vi "Open Project Reference.vi"(8 "error in (no error)":errorcluster, 10 "Path":path, 11 "App Ref":refnum<vi>) -> (0 "error out":errorcluster, 2 "VI Server Configured?":bool, 3 "App Ref out":refnum<vi>)   [LabVIEW 2020, in "MacroAssert.lvlib"]
doc: "Opens and outputs an application reference to a development system application instance that is owned by the project at <B>Path</B>."
uses:
  MacroAssert.lvlib
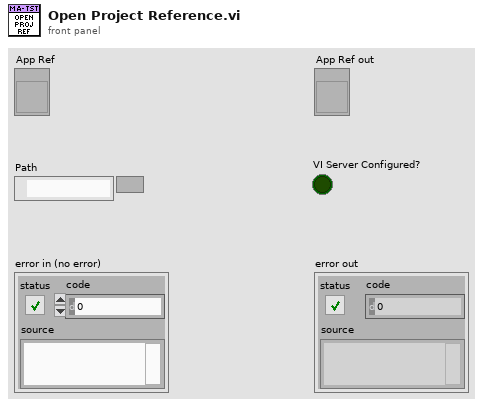
[diagram p1: front panel]
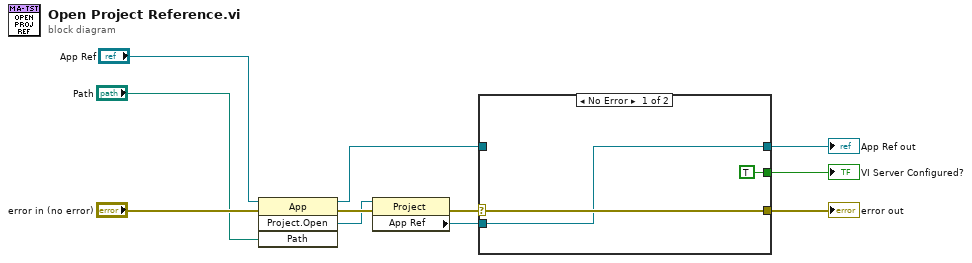
[diagram p0: block diagram]
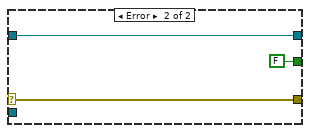
[diagram p2: hidden frame]
diagram:
  n1 = invoke class="App" method="Project.Open"(reference="App Ref", error in="error in (no error)", "Path"="Path") -> (reference out=w3:refnum<vi>, error out=w11:errorcluster, "Project:Open"=w7:refnum<vi>)  [unwired: 1 in, 1 out]
  n2 = property class="Project"(reference=w7, error in=w11) -> (error out=w9:errorcluster, "App Ref"=w4:refnum<vi>)  [unwired: 1 out]
  n3 = case shown="No Error" w9 {
    selector: w9 -> [w14 w17]
    tunnel: [w14 w17] -> w8
    tunnel: [w13 w16] -> w5
    tunnel: w4 -> [w13 _]
    tunnel: w3 -> [_ w16]
    tunnel: [TRUE FALSE] -> w1
    frame No Error {
    }
    frame Error {
    }
  }
  "error out" <- w8
  "App Ref out" <- w5
  "VI Server Configured?" <- w1
